vi "Wash_stages_FGV.vi"(7 "Task":enum16{"Clear", "Set", "Get", "Next Step"}(ring), 8 "error in (no error)":errorcluster, 11 "Wash Options":T2) -> (0 "error out":errorcluster, 3 "Current Station":T1)   [LabVIEW 2020]
doc: "FGV that tracks what stage the car wash is in."
uses:
  Controls/Queue_Control.ctl
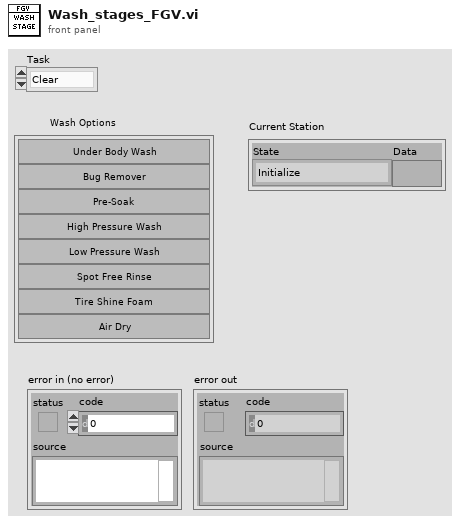
[diagram p1: front panel]
types:
  T1 = typedef "Queue_Control.ctl" = cluster{"State":enum16{"Initialize", "Start", "Next Station", "Under Body Wash", "Bug Remover", "Pre-soak", "High Pressure Wash", "Low Pressure Wash", "Spot Free Rinse", "Tire Shine Foam", "Air Dry", "Exit", "Check Position", "Out of Position", "Stop"}, "Data":variant}
  T2 = cluster{"Under Body Wash":bool, "Bug remover":bool, "Pre-soak":bool, "High Pressure Wash":bool, "Low Pressure Wash":bool, "Spot Free Rinse":bool, "Tire Shine Foam":bool, "Air Dry":bool}
  T3 = cluster{"Stations":enum16{"Under Body Wash", "Bug Remover", "Pre-soak", "High Pressure Wash", "Low Pressure Wash", "Spot Free Rinse", "Tire Shine Foam", "Air Dry", "Exit"}, "Time":u32}[]
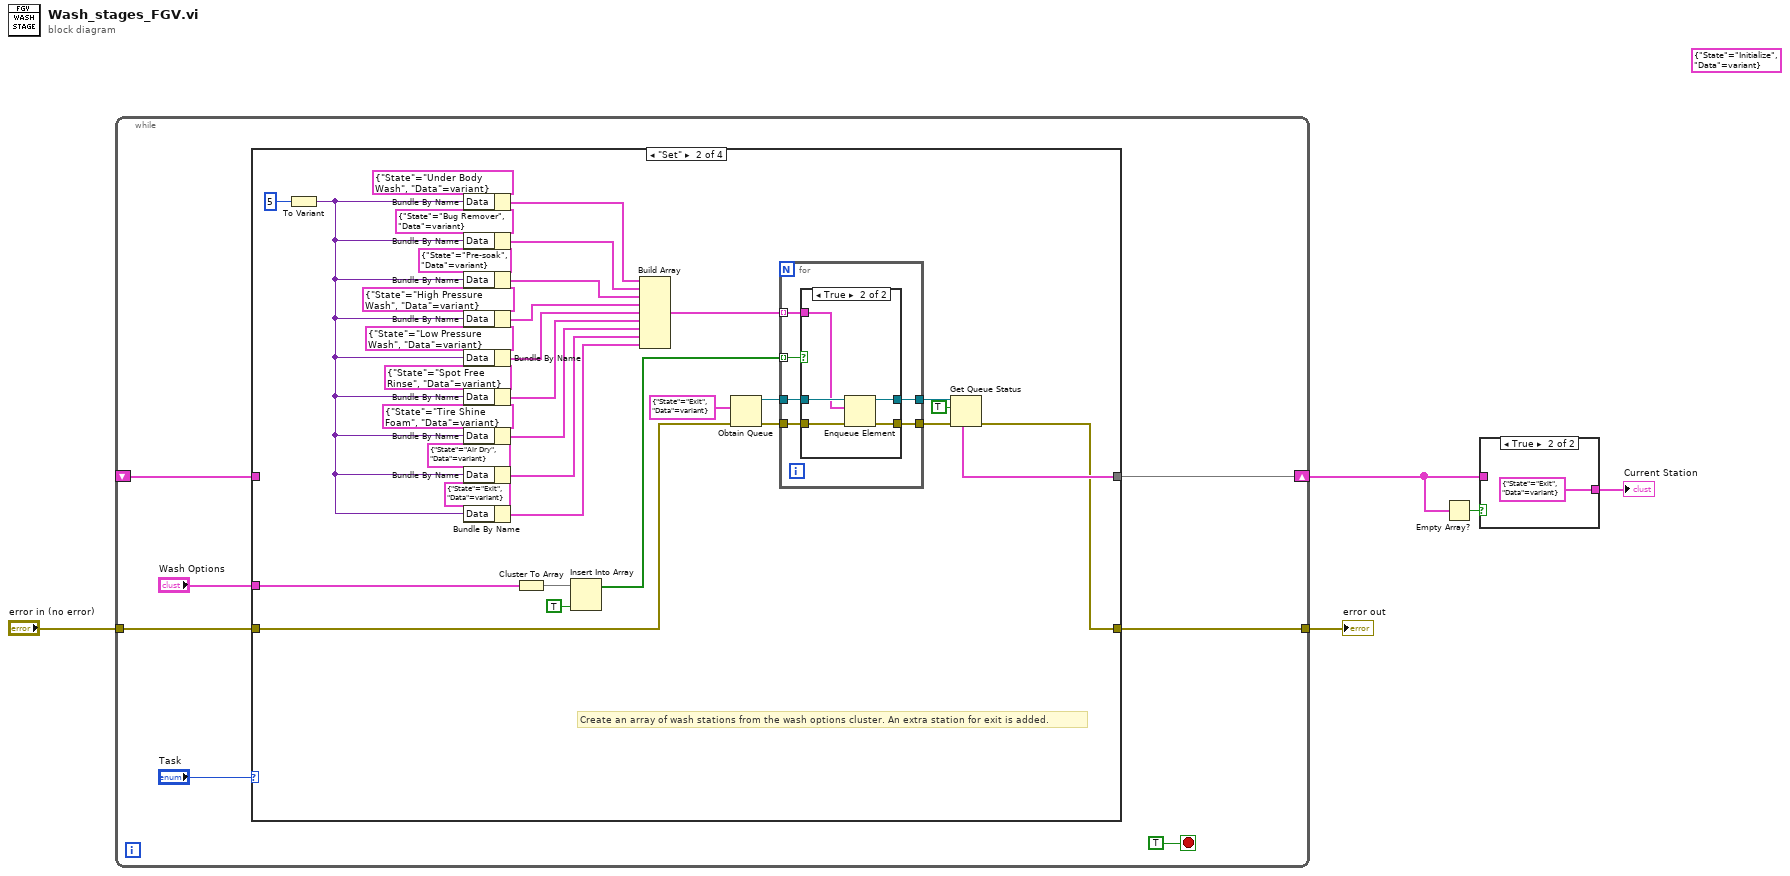
[diagram p0: block diagram]
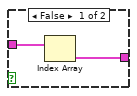
[diagram p2: hidden frame]
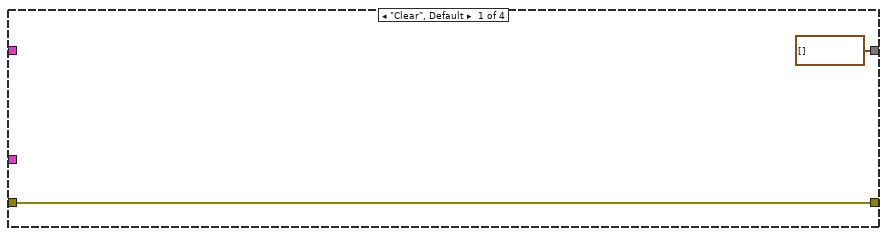
[diagram p3: hidden frame]
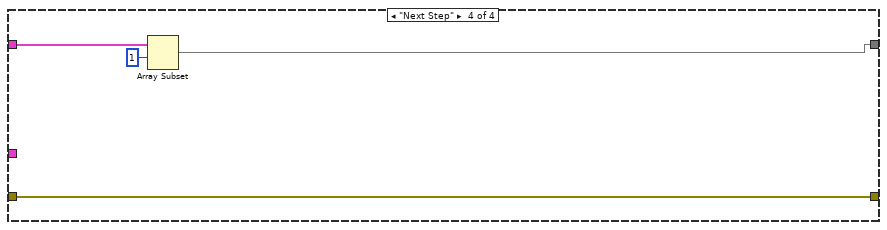
[diagram p6: hidden frame]
diagram:
  (unwired) T1 {"State"=enum."Initialize", "Data"=variant} ("Queue Control")
  n1 = while {
    shift-right: [w10] -> w2
    shift-left: _ -> [w7]
    tunnel: "error in (no error)" -> [w9]
    tunnel: [w8] -> w4
    stop <- TRUE stop-if-true
    n2 = case shown="\"Set\"" "Task" {
      tunnel: "Wash Options" -> [_ w36 _ _]
      tunnel: [T3 [] w42 w62 w64] -> w10
      tunnel: w9 -> [w14 w41 w63 w67]
      tunnel: [w14 w40 w63 w67] -> w8
      tunnel: w7 -> [_ _ w62 w65]
      frame "Clear", Default {
      }
      frame "Set" {
        # "Create an array of wash stations from the wash options cluster. An extra station for exit is added."
        n3 = To Variant(anything=u32 5) -> (Variant=w24:variant)
        n4 = Bundle By Name(cluster=T1 {"State"=enum."Under Body Wash", "Data"=variant} ("Queue Control"), "Data"=w24) -> (w23:T1)
        n5 = Bundle By Name(cluster=T1 {"State"=enum."Bug Remover", "Data"=variant} ("Queue Control"), "Data"=w24) -> (w22:T1)
        n6 = Bundle By Name(cluster=T1 {"State"=enum."Pre-soak", "Data"=variant} ("Queue Control"), "Data"=w24) -> (w21:T1)
        n7 = Bundle By Name(cluster=T1 {"State"=enum."High Pressure Wash", "Data"=variant} ("Queue Control"), "Data"=w24) -> (w20:T1)
        n8 = Bundle By Name(cluster=T1 {"State"=enum."Low Pressure Wash", "Data"=variant} ("Queue Control"), "Data"=w24) -> (w19:T1)
        n9 = Bundle By Name(cluster=T1 {"State"=enum."Spot Free Rinse", "Data"=variant} ("Queue Control"), "Data"=w24) -> (w18:T1)
        n10 = Bundle By Name(cluster=T1 {"State"=enum."Tire Shine Foam", "Data"=variant} ("Queue Control"), "Data"=w24) -> (w17:T1)
        n11 = Bundle By Name(cluster=T1 {"State"=enum."Air Dry", "Data"=variant} ("Queue Control"), "Data"=w24) -> (w16:T1)
        n12 = Bundle By Name(cluster=T1 {"State"=enum."Exit", "Data"=variant} ("Queue Control"), "Data"=w24) -> (w15:T1)
        n13 = Cluster To Array(cluster=w36) -> (array=w39:bool[])
        n14 = Insert Into Array(array=w39, new element=TRUE ("new element/subarray")) -> (w37:bool[])  [unwired: 1 in]
        n15 = Build Array(w23, w22, w21, w20, w19, w18, w17, w16, w15) -> (w48:T1[])
        n16 = Obtain Queue(element data type=T1 {"State"=enum."Exit", "Data"=variant} ("Queue Control"), error in (no error)=w41) -> (queue out=w47:refnum<queue>, error out=w46:errorcluster)  [unwired: 3 in, 1 out]
        n17 = for {
          tunnel: w37 -> [w54] mode=indexing
          tunnel: w48 -> [w53] mode=indexing
          tunnel: w47 -> [w51]
          tunnel: w46 -> [w52]
          tunnel: [w50] -> w45
          tunnel: [w49] -> w44
          n18 = case shown="True" w54 {
            tunnel: w53 -> [_ w57]
            tunnel: w52 -> [w55 w60]
            tunnel: w51 -> [w56 w61]
            tunnel: [w56 w59] -> w50
            tunnel: [w55 w58] -> w49
            frame False {
            }
            frame True {
              n19 = Enqueue Element(queue=w61, element=w57, error in (no error)=w60) -> (queue out=w59:refnum<queue>, error out=w58:errorcluster)  [unwired: 1 in, 1 out]
            }
          }
        }
        n20 = Get Queue Status(queue=w45, return elements? (F)=TRUE, error in (no error)=w44) -> (error out=w40:errorcluster, elements=w42:T1[])  [unwired: 6 out]
      }
      frame "Get" {
      }
      frame "Next Step" {
        n21 = Array Subset(array=w65, index=1) -> (w64:cluster{"State":u16, "Data":variant}[])  [unwired: 1 in]
      }
    }
  }
  "error out" <- w4
  n22 = Empty Array?(array=w2) -> (empty?=w3:bool)
  n23 = case shown="True" w3 {
    tunnel: w2 -> [w69 _]
    tunnel: [w68 T1 {"State"=enum."Exit", "Data"=variant} ("Queue Control")] -> w1
    frame False {
      n24 = Index Array(array=w69) -> (element=w68:cluster{"State":u16, "Data":variant})  [unwired: 1 in]
    }
    frame True {
    }
  }
  "Current Station" <- w1
